vi "acq_eeg_ini.vi"(8 "error in (no error)":errorcluster, 11 "eeg_device in":T1) -> (0 "error out":errorcluster, 2 "Variant":variant)   [LabVIEW 2013]
doc: "Opens the communication with the EEG device, based on its hardware"
uses:
  <vilib>/NIOSC/Address Space Node.ctl
  gui/type_def/device.ctl
  <vilib>/OpenBCI/Comm Protocol/Control Def/channel_count.ctl
  gui/type_def/file_stream.ctl
  gui/global_var.vi
  <vilib>/NI/Emotiv Toolkit/Emotiv Create Task Instances/EmoEngine.vi
  <vilib>/NI/Emotiv Toolkit/Emotiv Start Task Instances/Basic Start Task.vi
  <vilib>/NIOSC/NI_OSC.lvlib
  <vilib>/NI/Emotiv Toolkit/Emotiv Task.lvclass
  <vilib>/NI/LabVIEW - NeuroSky Driver/NeuroSky Driver.lvlib
panel:
  in  "muse cluster":T3
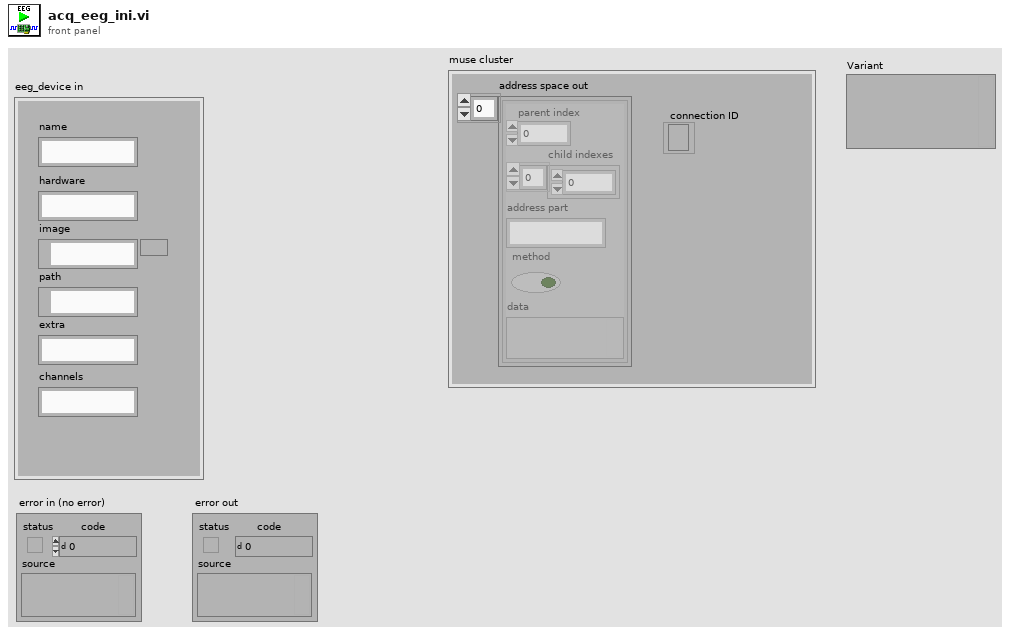
[diagram p1: front panel]
types:
  T1 = typedef "device.ctl" = cluster{"name":string, "hardware":string, "image":path, "path":path, "extra":string, "channels":string}
  T2 = typedef "NI_OSC.lvlib/Address Space Node.ctl" = cluster{"parent index":i32, "child indexes":i32[], "address part":string, "method":bool, "data":variant}
  T3 = cluster{"address space out":T2[], "connection ID":refnum<k5>}
  T4 = typedef "channel_count.ctl" = enum16{"8 Channels", "16 Channels"}
  T5 = typedef "file_stream.ctl" = cluster{"timestamp":timestamp, "data (2D array)":dbl[][], "Reading?":bool}
  T6 = cluster{"connectionId":i32, "serialPortName":string, "serialBaudrate":i32, "serialDataFormat":i32}
  T7 = typedef "openbci_device.ctl" = cluster{"COM port":refnum<visa-resource-name>, "n_ch (8)":T4, "delay_tx":u32}
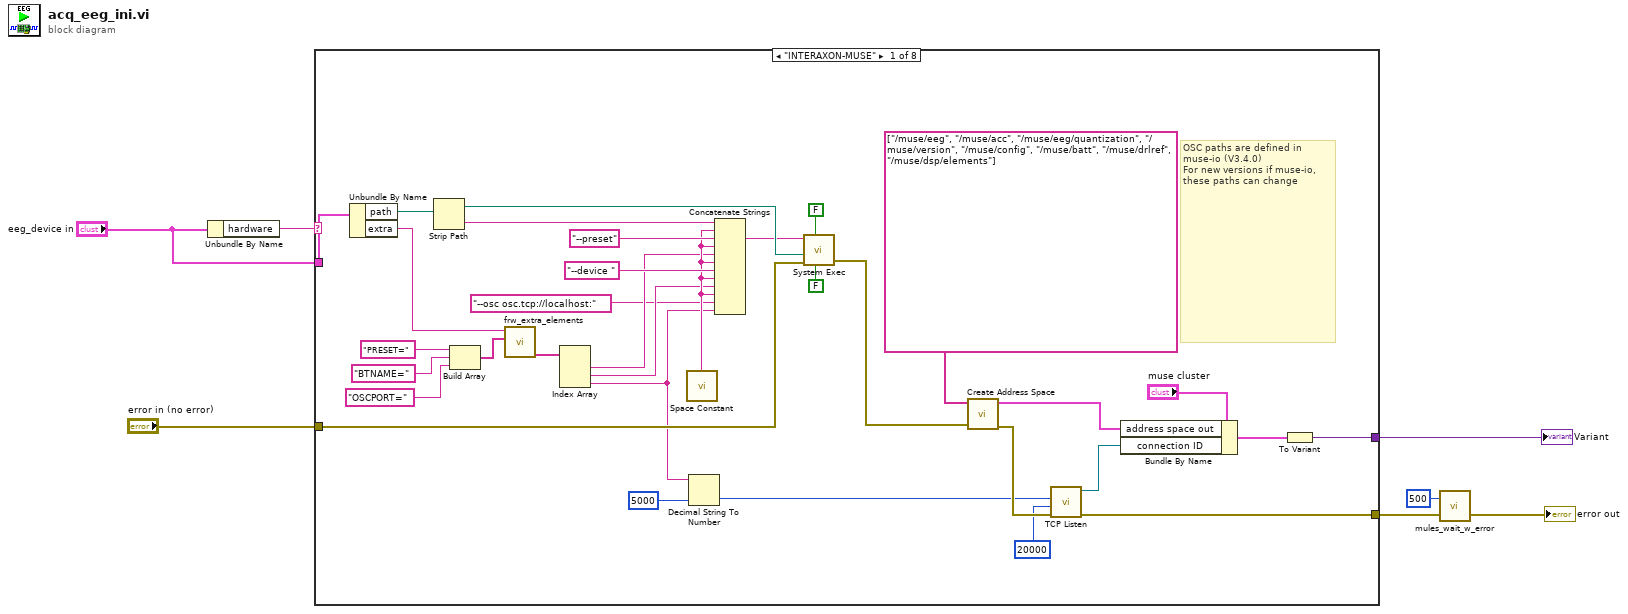
[diagram p0: block diagram]
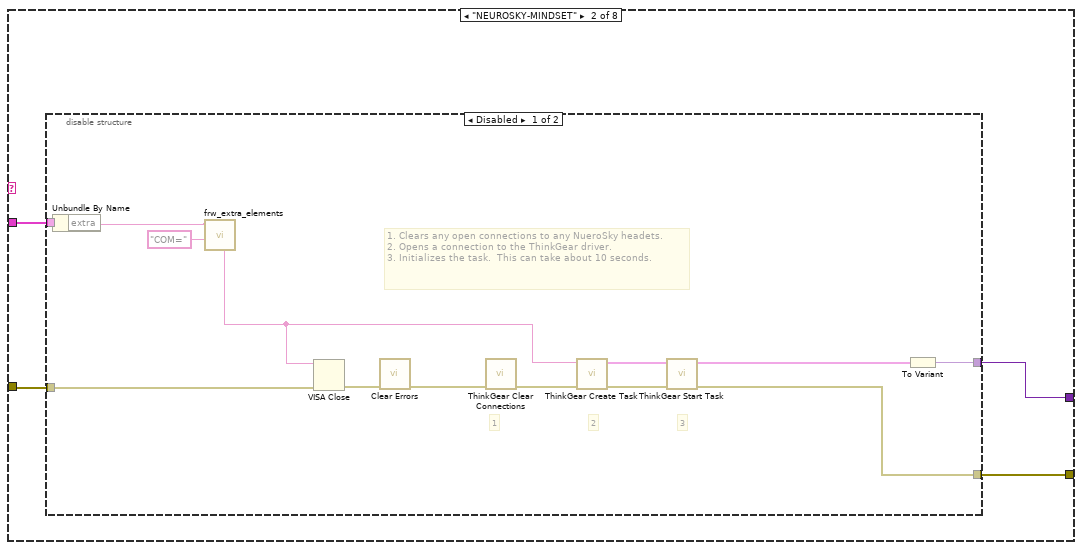
[diagram p2: hidden frame]
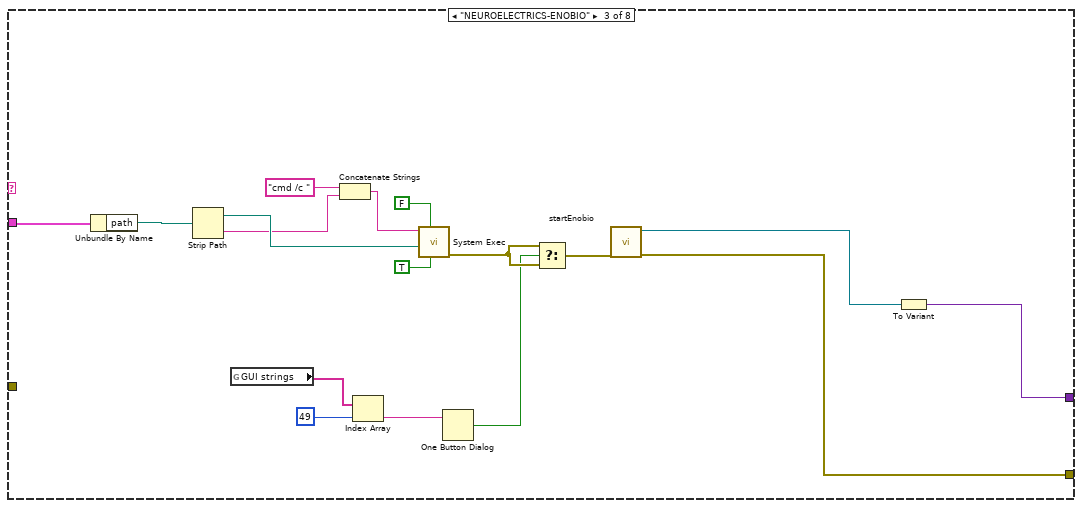
[diagram p4: hidden frame]
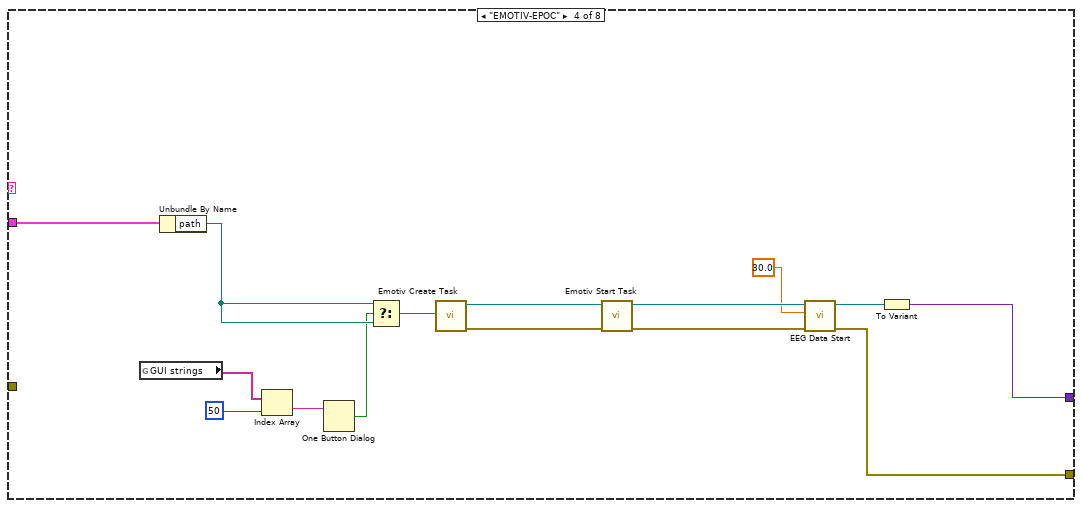
[diagram p5: hidden frame]
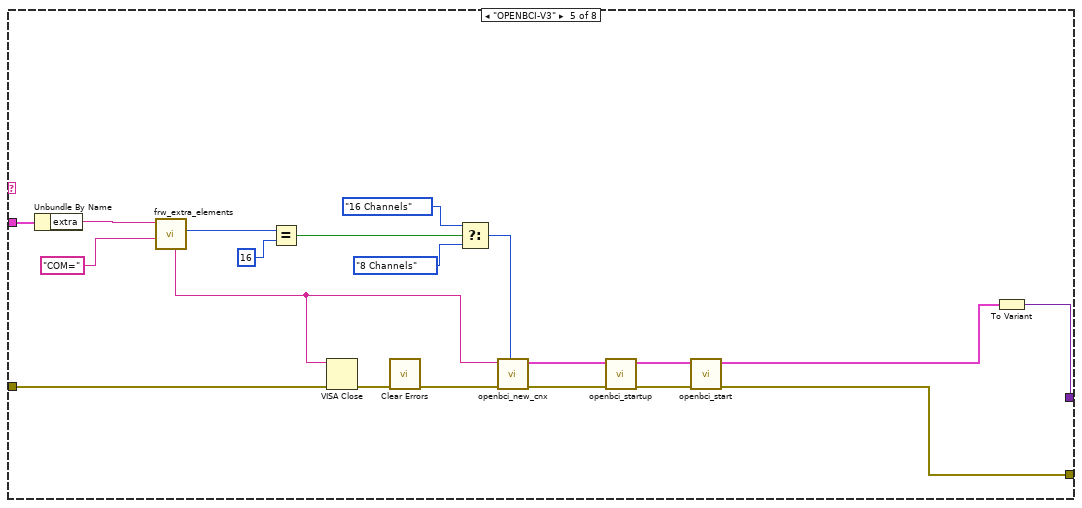
[diagram p6: hidden frame]
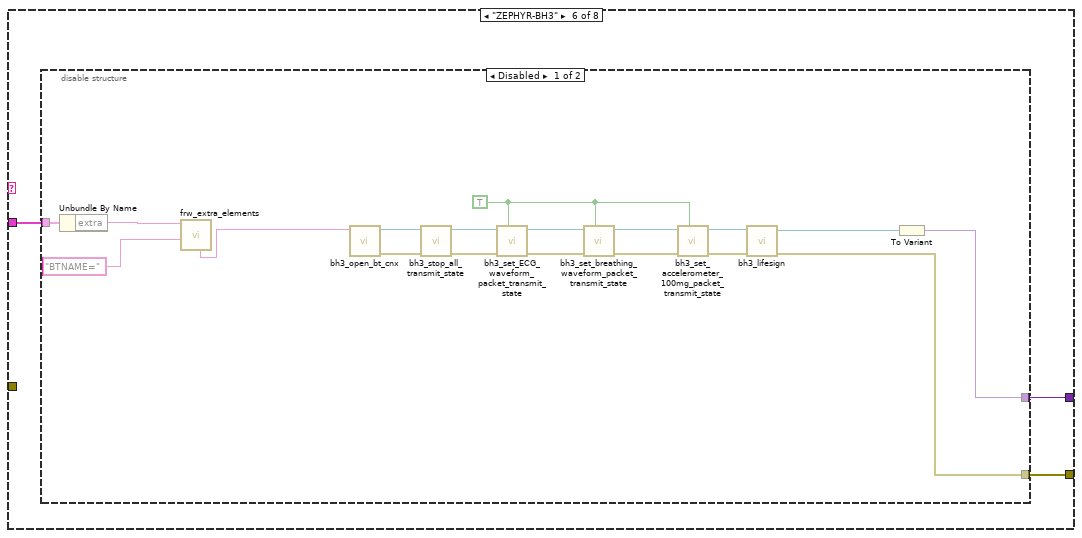
[diagram p7: hidden frame]
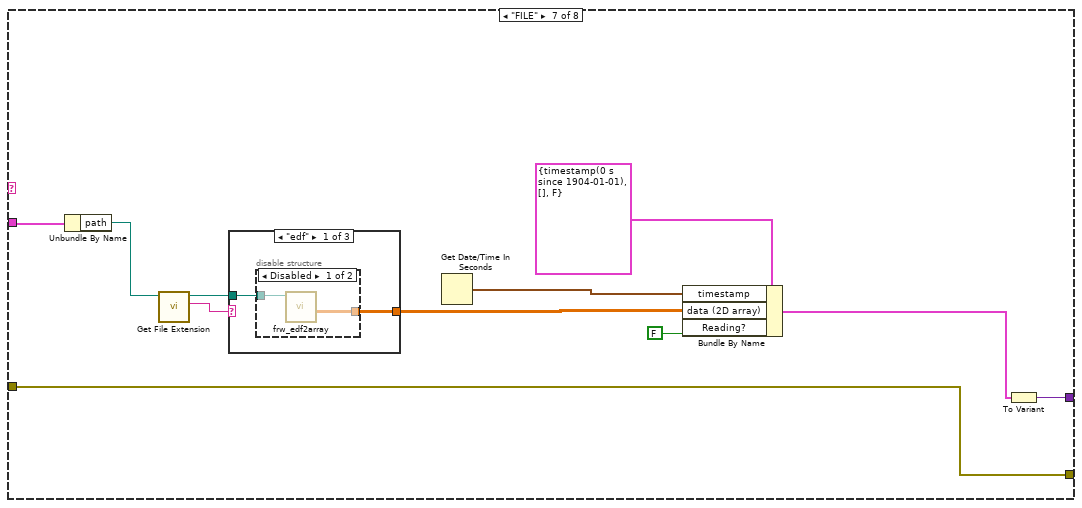
[diagram p9: hidden frame]
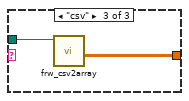
[diagram p12: hidden frame]
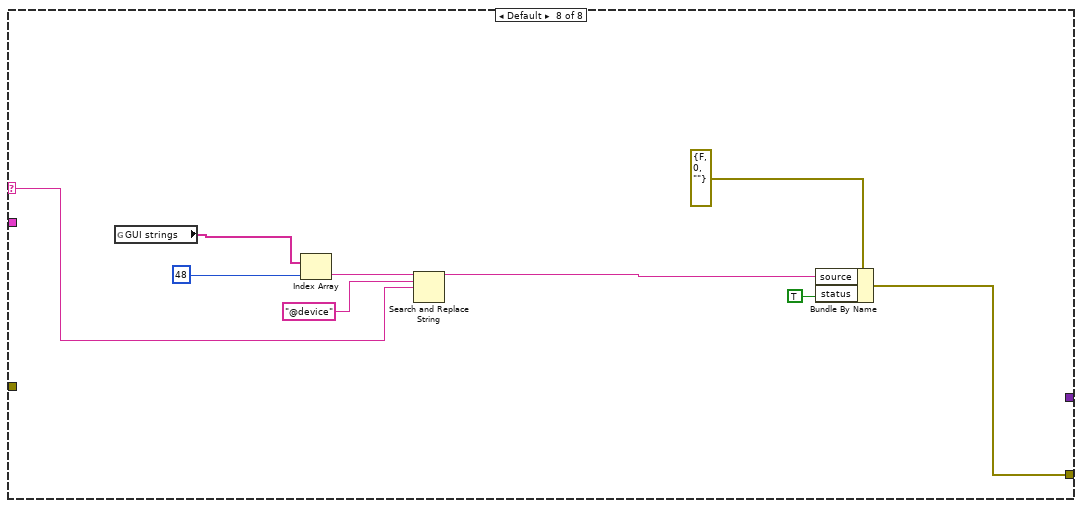
[diagram p13: hidden frame]
diagram:
  n1 = Unbundle By Name("eeg_device in") -> ("hardware"=w7:string)
  n2 = case shown="\"INTERAXON-MUSE\"" w7 {
    selector: w7 -> [_ _ _ _ _ _ _ w152]
    tunnel: "eeg_device in" -> [w40 w44 w74 w89 w109 w112 w139 _]
    tunnel: "error in (no error)" -> [w36 w41 _ _ w102 _ w141 _]
    tunnel: [w27 w43 w68 w83 w100 w110 w141 w150] -> w4
    tunnel: [w35 w42 w70 w82 w105 w111 w133 _] -> w5
    frame "INTERAXON-MUSE" {
      # "OSC paths are defined in muse-io (V3.4.0)\nFor new versions if muse-io, these paths can change"
      n3 = Unbundle By Name(w40) -> ("path"=w39:path, "extra"=w13:string)
      n4 = Strip Path(path=w39) -> (stripped path=w38:path, name=w24:string)
      n5 = Build Array("PRESET=" ("delimiter (Tab)"), "BTNAME=" ("delimiter (Tab)"), "OSCPORT=" ("delimiter (Tab)")) -> (w17:string[])
      n6 = call "frw_extra_elements.vi"("fields"=w17, "string"=w13) -> ("values"=w12:string[])  [unwired: 5 in, 4 out]
      n7 = Index Array(array=w12) -> (element #1=w11:string, element #2=w10:string, element #3=w8:string)  [unwired: 3 in]
      n8 = call <vilib>:"Space Constant.vi"() -> ("String"=w18:string)
      n9 = Decimal String To Number(string=w8, default (0L)=u16 5000 ("Local Port")) -> (number=w23:u16)  [unwired: 1 in, 1 out]
      n10 = Concatenate Strings(w24, w18, "--preset" ("string"), w18, w11, w18, "--device " ("string"), w18, w10, w18, "--osc osc.tcp://localhost:" ("string"), w8) -> (w26:string)
      n11 = call <vilib>:"System Exec.vi"("run minimized? (F)"=FALSE, "wait until completion? (T)"=FALSE, "error in (no error)"=w36, "working directory"=w38, "command line"=w26) -> ("error out"=w32:errorcluster)  [unwired: 3 in, 3 out]
      n12 = call <vilib>:"Create Address Space.vi"("error in"=w32, "method addresses"=string[] ["/muse/eeg", "/muse/acc", "/muse/eeg/quantization", "/muse/version", "/muse/config", "/muse/batt", "/muse/drlref", "/muse/dsp/elements"]) -> ("error out"=w33:errorcluster, "address space out"=w30:T2[])  [unwired: 8 in]
      n13 = call <vilib>:"TCP Listen.vi"("error in (no error)"=w33, "timeout ms (wait forever: -1)"=20000, "port"=w23) -> ("error out"=w27:errorcluster, "connection ID"=w29:refnum<k5>)  [unwired: 4 in, 3 out]
      n14 = Bundle By Name(cluster="muse cluster", "address space out"=w30, "connection ID"=w29) -> (w28:T3)
      n15 = To Variant(anything=w28) -> (Variant=w35:variant)
    }
    frame "NEUROSKY-MINDSET" {
      n16 = disable-structure shown="Disabled" {
        disable-tunnel: w44 -> [w54 _]
        disable-tunnel: [w53 _] -> w43
        disable-tunnel: [w52 _] -> w42
        disable-tunnel: w41 -> [w49 _]
        frame Disabled {
          # "1. Clears any open connections to any NueroSky headets.\n2. Opens a connection to the ThinkGear driver.\n3. Initializes the task.  This can take about 10 seconds."
          # "1"
          # "3"
          # "2"
          n17 = Unbundle By Name(w54) -> ("extra"=w47:string)
          n18 = call "frw_extra_elements.vi"("single field"="COM=", "string"=w47) -> ("single string"=w45:string)  [unwired: 5 in, 4 out]
          n19 = VISA Close(VISA resource name=w45, error in (no error)=w49) -> (error out=w50:errorcluster)
          n20 = call <vilib>:"Clear Errors.vi"("error in (no error)"=w50) -> ("error out"=w48:errorcluster)  [unwired: 6 in]
          n21 = call <vilib>:"ThinkGear Clear Connections.vi"("error in (no error)"=w48) -> ("error out"=w55:errorcluster)  [unwired: 10 in]
          n22 = call <vilib>:"ThinkGear Create Task.vi"("error in"=w55, "serialPortName"=w45) -> ("error out"=w56:errorcluster, "NeuroSky Task Out"=w57:T6)  [unwired: 8 in]
          n23 = call <vilib>:"ThinkGear Start Task.vi"("error in (no error)"=w56, "NeuroSky Task In"=w57) -> ("error out"=w53:errorcluster, "NeuroSky Task Out"=w51:T6)  [unwired: 8 in]
          n24 = To Variant(anything=w51) -> (Variant=w52:variant)
        }
        frame Enabled {
        }
      }
    }
    frame "NEUROELECTRICS-ENOBIO" {
      n25 = Unbundle By Name(w74) -> ("path"=w73:path)
      n26 = Strip Path(path=w73) -> (stripped path=w72:path, name=w63:string)
      n27 = global read "global_var.vi" "GUI strings"() -> (w60:string[])
      n28 = Concatenate Strings("cmd /c " ("string"), w63) -> (w62:string)
      n29 = Index Array(array=w60, index=49) -> (element=w58:string)
      n30 = call <vilib>:"System Exec.vi"("run minimized? (F)"=TRUE, "wait until completion? (T)"=FALSE, "working directory"=w72, "command line"=w62) -> ("error out"=w66:errorcluster)  [unwired: 4 in, 3 out]
      n31 = One Button Dialog(message=w58) -> (true=w65:bool)  [unwired: 1 in]
      n32 = Select(t=w66, s=w65, f=w66) -> (s? t:f=w67:errorcluster)
      n33 = call "startEnobio.vi"("error in (no error)"=w67) -> ("error out"=w68:errorcluster, "connection ID"=w69:refnum<k5>)  [unwired: 9 in]
      n34 = To Variant(anything=w69) -> (Variant=w70:variant)
    }
    frame "EMOTIV-EPOC" {
      n35 = global read "global_var.vi" "GUI strings"() -> (w77:string[])
      n36 = Unbundle By Name(w89) -> ("path"=w79:path)
      n37 = Index Array(array=w77, index=50) -> (element=w75:string)
      n38 = One Button Dialog(message=w75) -> (true=w78:bool)  [unwired: 1 in]
      n39 = Select(t=w79, s=w78, f=w79) -> (s? t:f=w80:path)
      n40 = call-poly <vilib>:"Emotiv Create Task.vi"("edk.dll Path"=w80) -> ("error out"=w88:errorcluster, "Emotiv Task out"=w87:refnum<class "Emotiv Task.lvclass">)  [unwired: 9 in]
      n41 = call-poly <vilib>:"Emotiv Start Task.vi"("error in (no error)"=w88, "Emotiv Task in"=w87) -> ("error out"=w86:errorcluster, "Emotiv Task out"=w85:refnum<class "Emotiv Task.lvclass">)  [unwired: 6 in]
      n42 = call <vilib>:"EEG Data Start.vi"("error in (no error)"=w86, "bufferSizeInSec"=sgl 30.0 ("BufferSize Emotive (sec)"), "Emotiv Task in"=w85) -> ("error out"=w83:errorcluster, "Emotiv Task out"=w81:refnum<class "Emotiv Task.lvclass">)  [unwired: 7 in]
      n43 = To Variant(anything=w81) -> (Variant=w82:variant)
    }
    frame "OPENBCI-V3" {
      n44 = Unbundle By Name(w109) -> ("extra"=w95:string)
      n45 = call "frw_extra_elements.vi"("single field"="COM=" ("delimiter (Tab)"), "string"=w95) -> ("fs"=w94:i32, "single string"=w90:string)  [unwired: 5 in, 3 out]
      n46 = Equal?(x=w94, y=16) -> (x = y?=w92:bool)
      n47 = VISA Close(VISA resource name=w90, error in (no error)=w102) -> (error out=w97:errorcluster)
      n48 = call <vilib>:"Clear Errors.vi"("error in (no error)"=w97) -> ("error out"=w96:errorcluster)  [unwired: 6 in]
      n49 = Select(t=channel_count."16 Channels" ("channel_count(8)"), s=w92, f=channel_count."8 Channels" ("channel_count(8)")) -> (s? t:f=w106:T4)
      n50 = call <vilib>:"openbci_new_cnx.vi"("channel_count(8)"=w106, "error in (no error)"=w96, "COM port"=w90) -> ("error out"=w103:errorcluster, "OBCI dev out"=w104:T7)  [unwired: 7 in]
      n51 = call <vilib>:"openbci_startup.vi"("error in"=w103, "OBCI dev in"=w104) -> ("error out"=w101:errorcluster, "OBCI dev out"=w99:T7)  [unwired: 7 in, 1 out]
      n52 = call <vilib>:"openbci_start.vi"("error in (no error)"=w101, "OBCI dev in"=w99) -> ("error out"=w100:errorcluster, "OBCI dev out"=w98:T7)  [unwired: 8 in]
      n53 = To Variant(anything=w98) -> (Variant=w105:variant)
    }
    frame "ZEPHYR-BH3" {
      n54 = disable-structure shown="Disabled" {
        disable-tunnel: w112 -> [w128 _]
        disable-tunnel: [w114 _] -> w111
        disable-tunnel: [w113 _] -> w110
        frame Disabled {
          w116 = TRUE ("enable?")
          n55 = Unbundle By Name(w128) -> ("extra"=w130:string)
          n56 = call "frw_extra_elements.vi"("single field"="BTNAME=" ("delimiter (Tab)"), "string"=w130) -> ("single string"=w127:string)  [unwired: 5 in, 4 out]
          n57 = call <vilib>:"bh3_open_bt_cnx.vi"("device name"=w127) -> ("error out"=w117:errorcluster, "bt connection ID"=w126:refnum<k31>)  [unwired: 9 in]
          n58 = call <vilib>:"bh3_stop_all_transmit_state.vi"("error in (no error)"=w117, "bt connection ID in"=w126) -> ("error out"=w118:errorcluster, "bt connection ID out"=w125:refnum<k31>)  [unwired: 8 in]
          n59 = call <vilib>:"bh3_set_ECG_waveform_packet_transmit_state.vi"("enable?"=w116, "error in (no error)"=w118, "bt connection ID in"=w125) -> ("error out"=w119:errorcluster, "bt connection ID out"=w124:refnum<k31>)  [unwired: 7 in]
          n60 = call <vilib>:"bh3_set_breathing_waveform_packet_transmit_state.vi"("enable?"=w116, "error in (no error)"=w119, "bt connection ID in"=w124) -> ("error out"=w120:errorcluster, "bt connection ID out"=w123:refnum<k31>)  [unwired: 7 in]
          n61 = call <vilib>:"bh3_set_accelerometer_100mg_packet_transmit_state.vi"("enable?"=w116, "error in (no error)"=w120, "bt connection ID in"=w123) -> ("error out"=w121:errorcluster, "bt connection ID out"=w122:refnum<k31>)  [unwired: 7 in]
          n62 = call <vilib>:"bh3_lifesign.vi"("error in (no error)"=w121, "bt connection ID in"=w122) -> ("error out"=w113:errorcluster, "bt connection ID out"=w115:refnum<k31>)  [unwired: 8 in]
          n63 = To Variant(anything=w115) -> (Variant=w114:variant)
        }
        frame Enabled {
        }
      }
    }
    frame "FILE" {
      n64 = Unbundle By Name(w139) -> ("path"=w135:path)
      n65 = call <vilib>:"Get File Extension.vi"("file"=w135) -> ("lowercase file extension"=w140:string, "dup file"=w134:path)  [unwired: 7 in, 2 out]
      n66 = case shown="\"edf\"" w140 {
        tunnel: w134 -> [w143 _ w147]
        tunnel: [w142 _ w146] -> w136
        frame "edf" {
          n67 = disable-structure shown="Disabled" {
            disable-tunnel: w143 -> [w145 _]
            disable-tunnel: [w144 _] -> w142
            frame Disabled {
              n68 = call "frw_edf2array.vi"("file path"=w145) -> ("2D array"=w144:dbl[][])  [unwired: 8 in, 2 out]
            }
            frame Enabled {
            }
          }
        }
        frame Default {
        }
        frame "csv" {
          n69 = call "frw_csv2array.vi"("file path"=w147) -> ("values"=w146:dbl[][])  [unwired: 7 in, 3 out]
        }
      }
      n70 = Get Date/Time In Seconds() -> (seconds since 1Jan1904=w137:timestamp)
      n71 = Bundle By Name(cluster=T5 {"timestamp"=timestamp(0 s since 1904-01-01), "data (2D array)"=[], "Reading?"=FALSE} ("output cluster"), "timestamp"=w137, "data (2D array)"=w136, "Reading?"=FALSE) -> (w132:T5)
      n72 = To Variant(anything=w132) -> (Variant=w133:variant)
    }
    frame Default {
      n73 = global read "global_var.vi" "GUI strings"() -> (w154:string[])
      n74 = Index Array(array=w154, index=48) -> (element=w155:string)
      n75 = Search and Replace String(input string=w155, search string="@device", replace string=w152) -> (result string=w149:string)  [unwired: 5 in, 3 out]
      n76 = Bundle By Name(cluster=errorcluster {"status"=FALSE, "code"=0, "source"=""} ("error constant"), "source"=w149, "status"=TRUE) -> (w150:errorcluster)
    }
  }
  "Variant" <- w5
  n77 = call "mules_wait_w_error.vi"("error in (no error)"=w4, "milliseconds to wait"=u32 500) -> ("error out"=→"error out":errorcluster)  [unwired: 1 in]
